vi "Keithley 2600 Series Read Pulsed Voltage Measurement.vi"() -> ()   [LabVIEW 2011]
doc: "This example shows how to configure a pulsed current with voltage measurement."
uses:
  <instrlib>/Keithley 2600 Series/Public/Configure/Source/Configure Source (Limit).vi
  <instrlib>/Keithley 2600 Series/Keithley 2600 Series.lvlib
panel:
  in  "Voltage Limit (5 V)":dbl=5.0
  out "Voltage (V)":dbl[](array[numeric])
  in  "VISA resource name":refnum<visa-resource-name>
  in  "Sweep Points (10)":i32=10
  in  "Pulse Off Time (0.4 S)":dbl=0.4
  in  "Pulse On Time (0.2 S)":dbl=0.2
  in  "Pulse Level (0.1 A)":dbl=0.1
  in  "Bias Level (0.001 A)":dbl=0.001
  in  "Source Measure Unit Channel (0: Channel A)":i32(ring) items=["Channel A", "Channel B"]
  # "(c) 2020 National Instruments.  ALL RIGHTS RESERVED."
  # "Current Pulse Configuration"
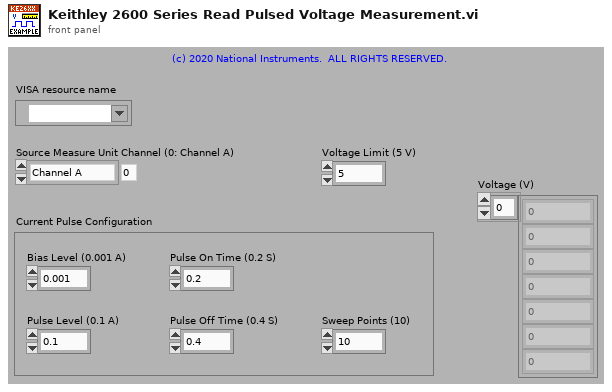
[diagram p1: front panel]
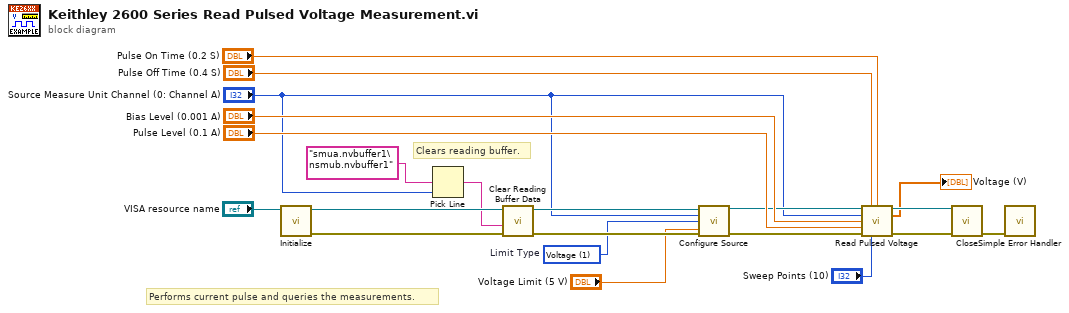
[diagram p0: block diagram]
diagram:
  w6 = 1 items=["Current", "Voltage", "Power"]  # Limit Type
  # "Performs current pulse and queries the measurements."
  # "Clears reading buffer."
  n1 = call <instrlib>:"Initialize.vi"("VISA resource name"="VISA resource name") -> ("error out"=w2:errorcluster, "VISA resource name out"=w3:refnum<visa-resource-name>)  [unwired: 9 in]
  n2 = Pick Line(multi-line string="smua.nvbuffer1\nsmub.nvbuffer1", line index="Source Measure Unit Channel (0: Channel A)") -> (output string=w1:string)  [unwired: 1 in]
  n3 = call <instrlib>:"Clear Reading Buffer Data.vi"("error in (no error)"=w2, "Reading Buffer (smua.nvbuffer1)"=w1, "VISA resource name"=w3) -> ("error out"=w15:errorcluster, "VISA resource name out"=w16:refnum<visa-resource-name>)  [unwired: 7 in]
  n4 = call-poly <instrlib>:"Configure Source.vi"("VISA resource name"=w16, "Source Measure Unit Channel (0: Channel A)"="Source Measure Unit Channel (0: Channel A)", "Limit Type (1: Voltage)"=w6, "error in (no error)"=w15, "Voltage Limit (20 V)"="Voltage Limit (5 V)") -> ("VISA resource name out"=w14:refnum<visa-resource-name>, "error out"=w13:errorcluster)  [unwired: 9 in]
  n5 = call <instrlib>:"Read Pulsed Voltage.vi"("VISA resource name"=w14, "Pulse Off Time (0.4 S)"="Pulse Off Time (0.4 S)", "Pulse On Time (0.2 S)"="Pulse On Time (0.2 S)", "Source Measure Unit Channel (0: Channel A)"="Source Measure Unit Channel (0: Channel A)", "Bias Level (0.001 A)"="Bias Level (0.001 A)", "Pulse Level (1 A)"="Pulse Level (0.1 A)", "error in (no error)"=w13, "Sweep Points (10)"="Sweep Points (10)") -> ("VISA resource name out"=w9:refnum<visa-resource-name>, "Voltage (V)"=→"Voltage (V)":dbl[], "error out"=w8:errorcluster)  [unwired: 5 in]
  n6 = call <instrlib>:"Close.vi"("error in (no error)"=w8, "VISA resource name"=w9) -> ("error out"=w11:errorcluster)  [unwired: 9 in]
  n7 = call <vilib>:"Simple Error Handler.vi"("error in (no error)"=w11) -> ()  [unwired: 4 in, 5 out]
